vi "ReadingLastLineInDataFile.vi"(0 "file path (dialog if empty)":path, 5 "error in (no error)":errorcluster) -> (6 "Channel 1 value 1":string, 7 "Channel 1 value 2":string, 8 "Channel 2 value 1":string, 9 "Channel 2 value 2":string, 10 "Channel 3 value 1":string, 11 "Channel 3 value 2":string, 12 "Channel 4 value 2":string, 13 "Channel 4 value 1":string, 14 "Array with data values":string[](array[string]), 19 "error out":errorcluster)   [LabVIEW 2020, in "ReadingDataFile.lvlib"]
uses:
  ReadingDataFile.lvlib
  <vilib>/Utility/file.llb/Read Delimited Spreadsheet (string).vi
panel:
  out "Last row":string[](array[string])
  out "Row size":i32
  out "Col size":i32
  out "all rows":string[][](array[string])
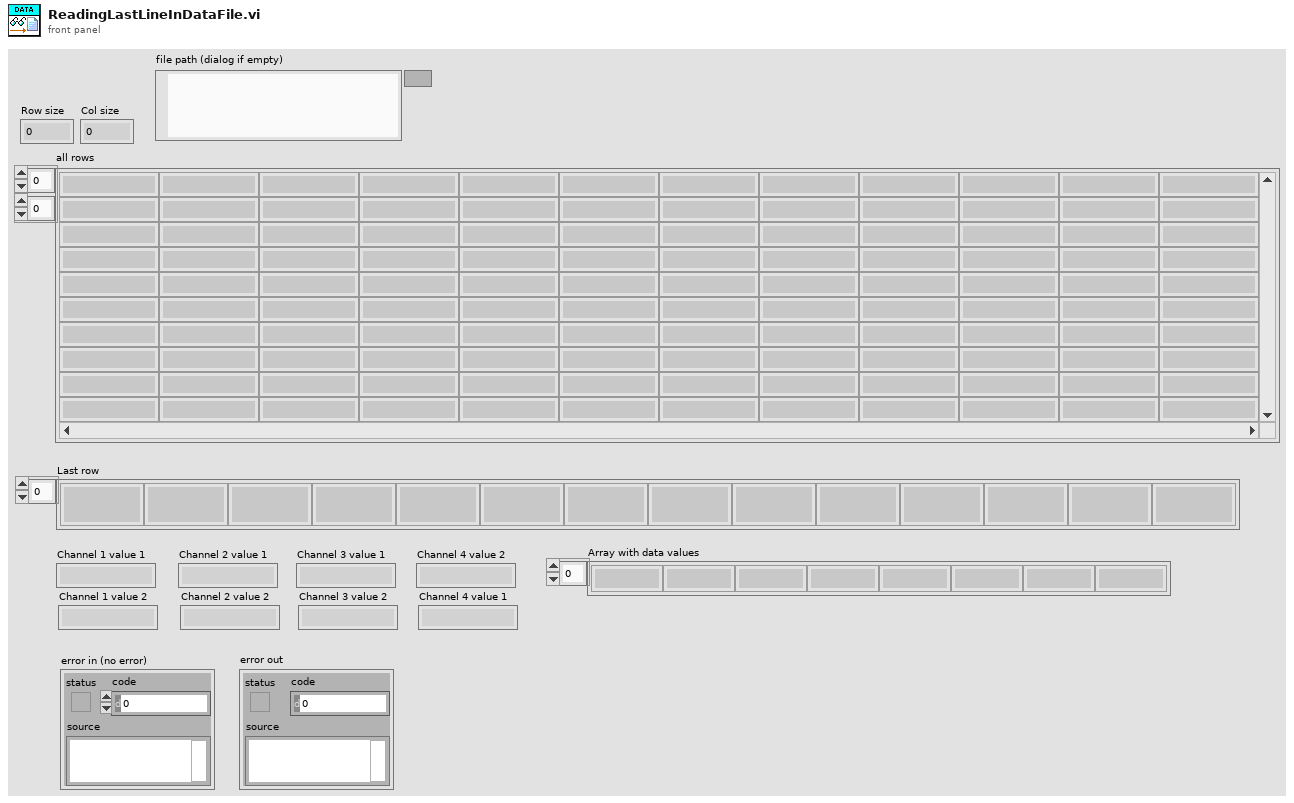
[diagram p1: front panel]
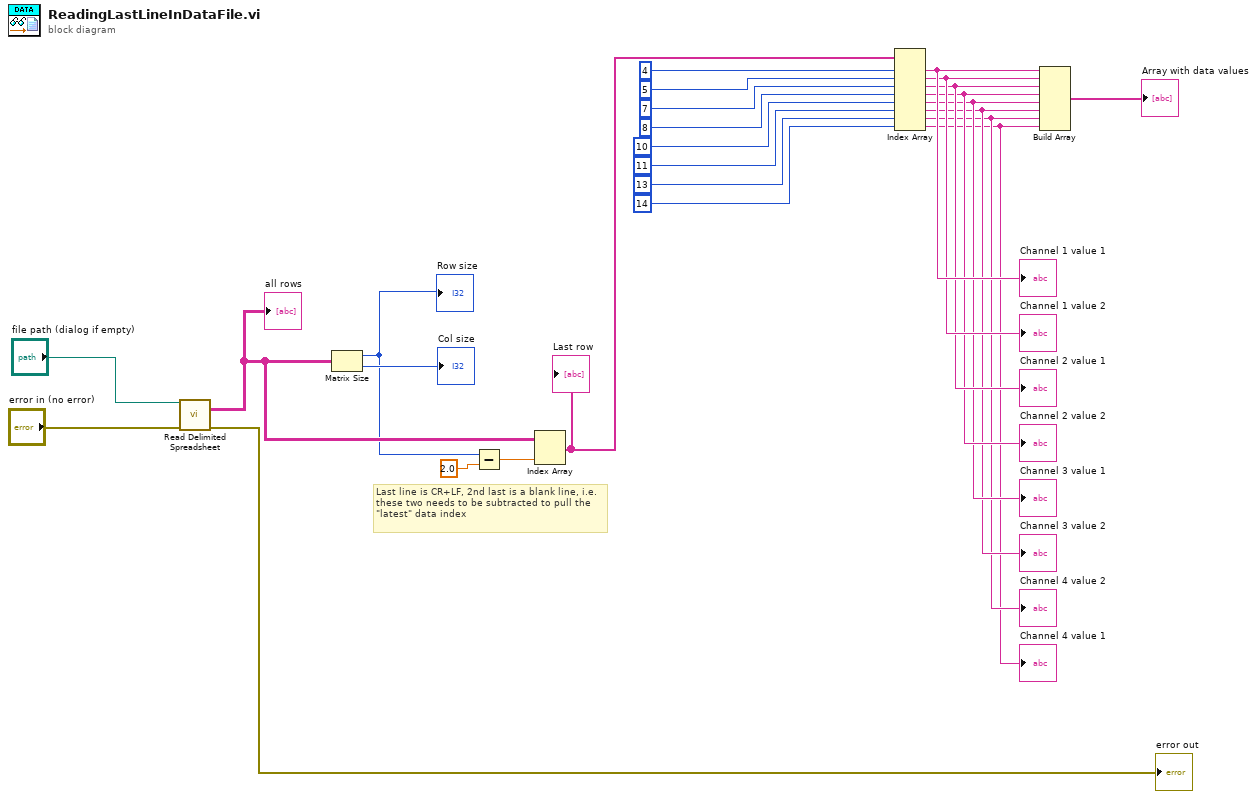
[diagram p0: block diagram]
diagram:
  # "Last line is CR+LF, 2nd last is a blank line, i.e. these two needs to be subtracted to pull the \"latest\" data index"
  n1 = call-poly <vilib>:"Read Delimited Spreadsheet.vi"("file path (dialog if empty)"="file path (dialog if empty)", "error in (no error)"="error in (no error)") -> ("all rows"=w24:string[][], "error out"=→"error out":errorcluster)  [unwired: 8 in, 4 out]
  "all rows" <- w24
  n2 = Matrix Size(0:w24) -> (1:w22:i32, 2:→"Col size":i32)
  "Row size" <- w22
  n3 = Subtract(x=w22, y=2.0) -> (x-y=w25:dbl)
  n4 = Index Array(array=w24, index (row)=w25) -> (element=w19:string[])  [unwired: 1 in]
  "Last row" <- w19
  n5 = Index Array(array=w19, index #1=4 ("index"), index #2=5 ("index"), index #3=7 ("index"), index #4=8 ("index"), index #5=10 ("index"), index #6=11 ("index"), index #7=13 ("index"), index #8=14 ("index")) -> (element #1=w10:string, element #2=w9:string, element #3=w8:string, element #4=w7:string, element #5=w6:string, element #6=w5:string, element #7=w4:string, element #8=w3:string)
  "Channel 1 value 1" <- w10
  "Channel 1 value 2" <- w9
  "Channel 2 value 1" <- w8
  "Channel 2 value 2" <- w7
  "Channel 3 value 1" <- w6
  "Channel 3 value 2" <- w5
  "Channel 4 value 2" <- w4
  "Channel 4 value 1" <- w3
  n6 = Build Array(w10, w9, w8, w7, w6, w5, w4, w3) -> (→"Array with data values":string[])
